vi "AcquireFixation.vi"(8 "error in (no error)":errorcluster, 11 "TrialBasedExperiment in":refnum<class "TrialBasedExperiment.lvclass">) -> (0 "error out":errorcluster, 2 "Timeout":dbl, 3 "TrialBasedExperiment out":refnum<class "TrialBasedExperiment.lvclass">)   [LabVIEW 2010, in "TrialBasedExperiment.lvclass"]
uses:
  TrialBasedExperiment.lvclass
  TrialBasedExperiment.lvclass/TrialBasedExperiment.ctl
  Acquisition/BehaviorData/BehaviorData.lvclass
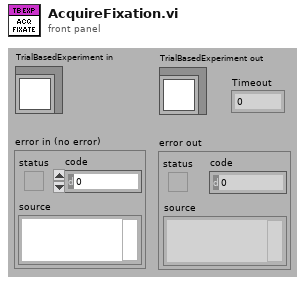
[diagram p1: front panel]
types:
  T1 = enum16{"Get Time", "Get Elapsed Time", "Reset Elapsed Time"}
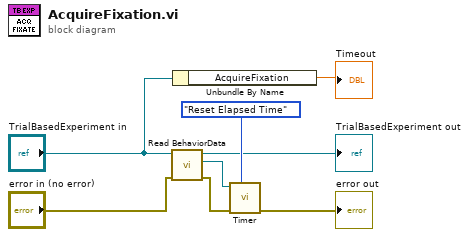
[diagram p0: block diagram]
diagram:
  n1 = call-dynamic "Read BehaviorData.vi"("error in (no error)"="error in (no error)", "TrialBasedExperiment in"="TrialBasedExperiment in") -> ("error out"=w6:errorcluster, "BehaviorData.lvclass"=w7:refnum<class "BehaviorData.lvclass">, "TrialBasedExperiment out"=→"TrialBasedExperiment out":refnum<class "TrialBasedExperiment.lvclass">)  [unwired: 7 in]
  n2 = Unbundle By Name("TrialBasedExperiment in") -> ("AcquireFixation"=→"Timeout":dbl)
  n3 = call-dynamic "Timer.vi"("Method"=T1."Reset Elapsed Time", "error in (no error)"=w6, "BehaviorData in"=w7) -> ("error out"=→"error out":errorcluster)  [unwired: 5 in, 3 out]
